vi "UI_Drive_Unit.vi"() -> ()   [LabVIEW 2014]
panel:
  out "GEAR_SYS_DATA":T1
  out "DRIVE_SYS_DATA":T2
  in  "退出":bool
  # "驱动单元监测参数"
  # "齿\n轮\n子\n系\n统"
  # "动\n力\n子\n系\n统"
  # "报警信息"
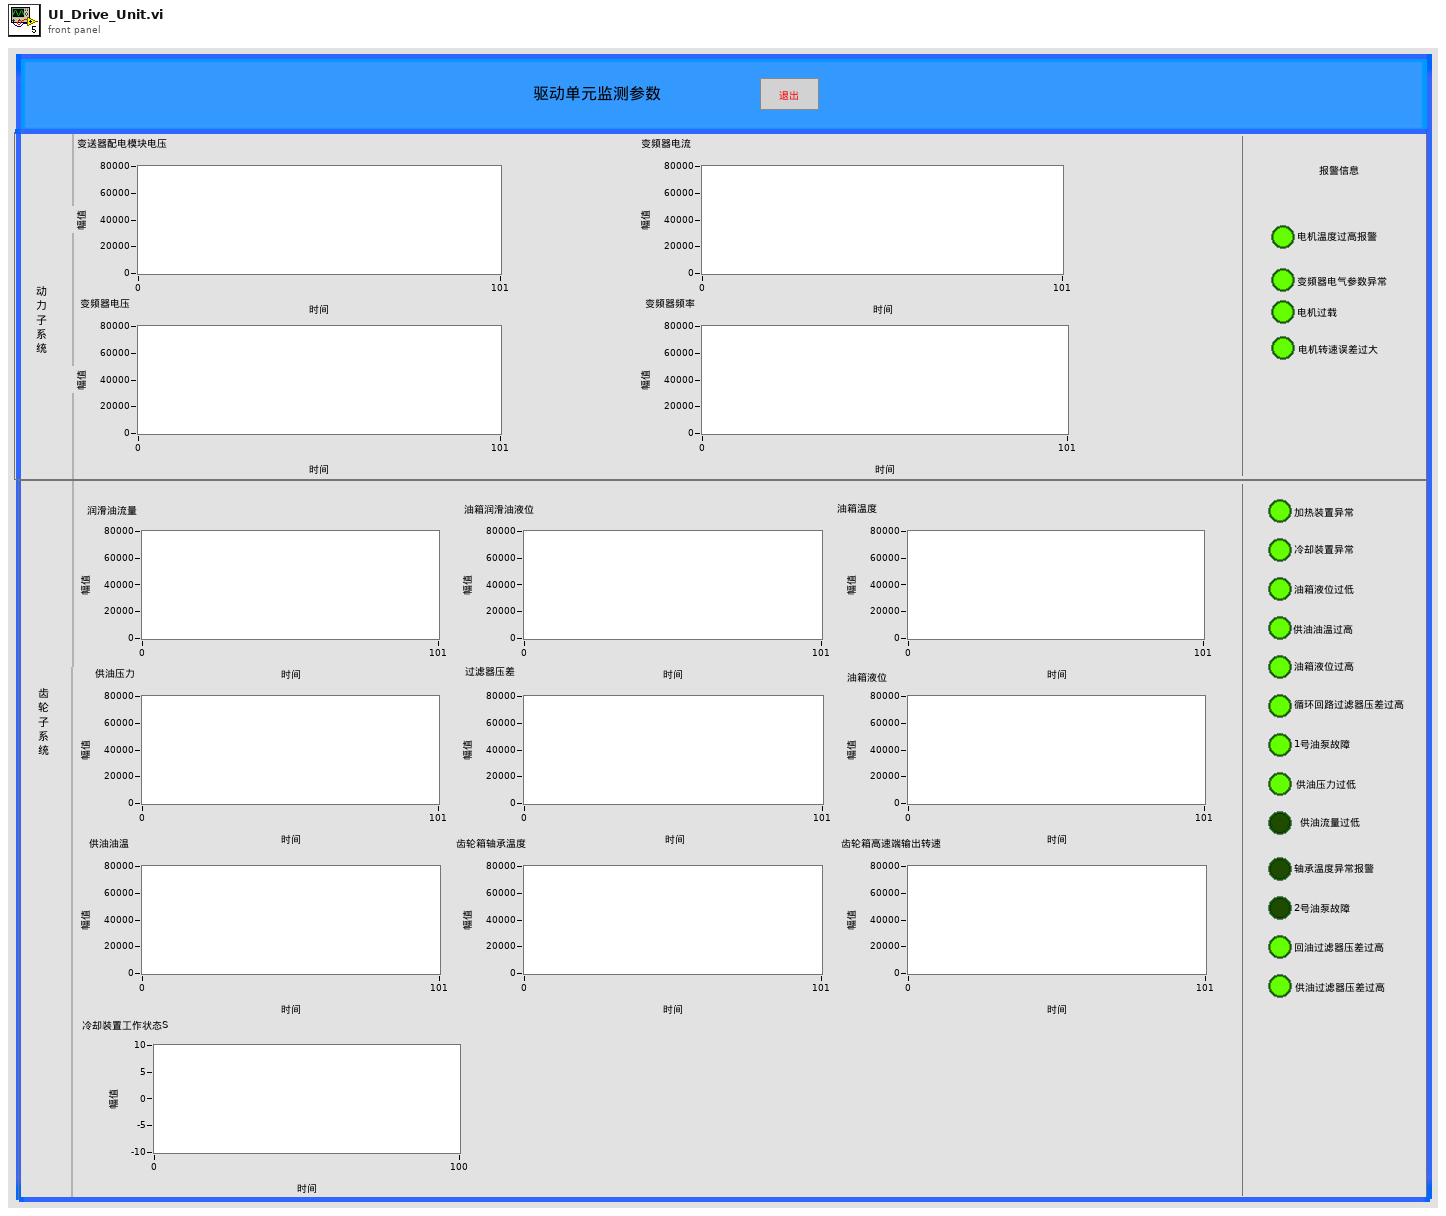
[diagram p1: front panel]
types:
  T1 = cluster{"润滑油流量":cluster{sgl, sgl, "润滑油流量":u16}, "油箱润滑油液位":cluster{sgl, sgl, "油箱润滑油液位":u16}, "油箱温度":cluster{sgl, sgl, "油箱温度":u16}, "冷却装置工作状态S":dbl, "径向液压缸加载压力 3":cluster{sgl, sgl, "供油压力":u16}, "过滤器压差":cluster{sgl, sgl, "过滤器压差":u16}, "油箱液位":cluster{sgl, sgl, "油箱液位":u16}, "供油油温":cluster{sgl, sgl, "供油油温":u16}, "齿轮箱轴承温度":cluster{sgl, sgl, "齿轮箱轴承温度":u16}, "齿轮箱高速端输出转速":cluster{sgl, sgl, "齿轮箱高速端输出转速":u16}, "齿轮子系统报警信息":cluster{"齿轮子系统加热装置异常":bool, "齿轮子系统冷却装置异常":bool, "齿轮子系统油箱液位过低":bool, "齿轮子系统供油油温过高":bool, "齿轮子系统油箱液位过高":bool, "齿轮子系统循环回路过滤器压差过高":bool, "齿轮子系统1号油泵故障":bool, "齿轮子系统供油压力过低":bool, "齿轮子系统供油流量过低":bool, "齿轮子系统轴承温度异常报警":bool, "齿轮子系统2号油泵故障":bool, "齿轮子系统回油过滤器压差过高":bool, "齿轮子系统供油过滤器压差过高":bool}}
  T2 = cluster{"变送器配电模块电压":cluster{sgl, sgl, "变送器配电模块电压":u16}, "变频器电流":cluster{sgl, sgl, "变频器电流":u16}, "变频器电压":cluster{sgl, sgl, "变频器电压":u16}, "变频器频率":cluster{sgl, sgl, "变频器频率":u16}, "动力子系统报警":cluster{"电机温度过高报警":bool, "动力子系统变频器电气参数异常":bool, "动力子系统电机过载":bool, "动力子系统电机转速误差过大":bool}}
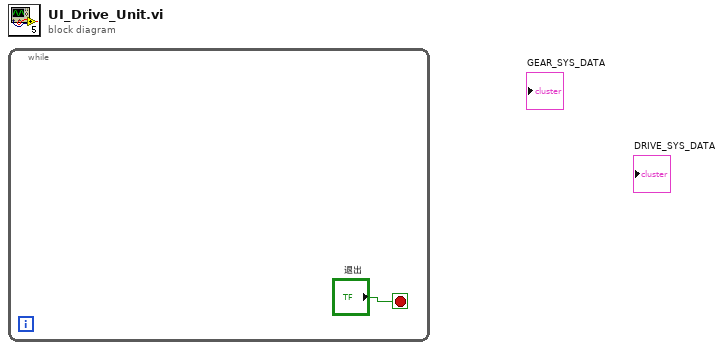
[diagram p0: block diagram]
diagram:
  n1 = while {
    stop <- "退出" stop-if-true
  }
